vi "Add Signals.vi"(0 "reference in":refnum<class "SigMath.lvclass">, 5 "error in (no error)":errorcluster, 7 "Select Signals":i32[](listbox)) -> (14 "reference out":refnum<class "SigMath.lvclass">, 19 "error out":errorcluster)   [LabVIEW 2020, in "SigMath.lvclass"]
uses:
  SigMath.lvclass
  API/GSwFormDSP_class/functions/Attribute List.ctl
  API/GSwFormDSP_class/functions/Attribute Options.ctl
  API/GSwFormDSP_class/GSwFormDSP.lvclass
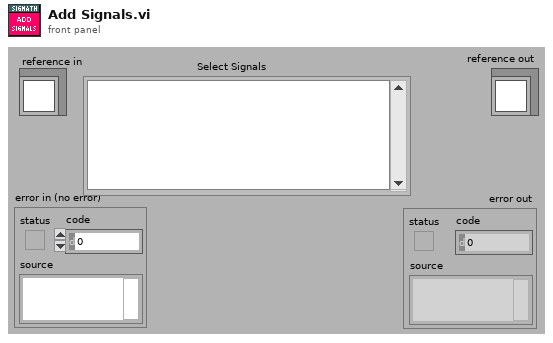
[diagram p1: front panel]
types:
  T1 = typedef "GSwFormDSP.lvclass/Attribute Options.ctl" = enum16{"Append to Attribute using \"( )\"", "Replace Attribute Value"}
  T2 = typedef "GSwFormDSP.lvclass/Attribute List.ctl" = string
  T3 = typedef "SigMath.lvclass/ObjectAttributes.ctl" = cluster{"SigMath Data":T4, "User CTRL Refs":T5}
  T4 = typedef "SigMath.lvclass/SigMath Data.ctl" = cluster{"New Time Data Obj?":bool, "GSwFormDSP":refnum<class "GSwFormDSP.lvclass">}
  T5 = typedef "SigMath.lvclass/SigMath User CTRL Refs.ctl" = cluster{"wForms":refnum<vi>, "Results wForms":refnum<vi>}
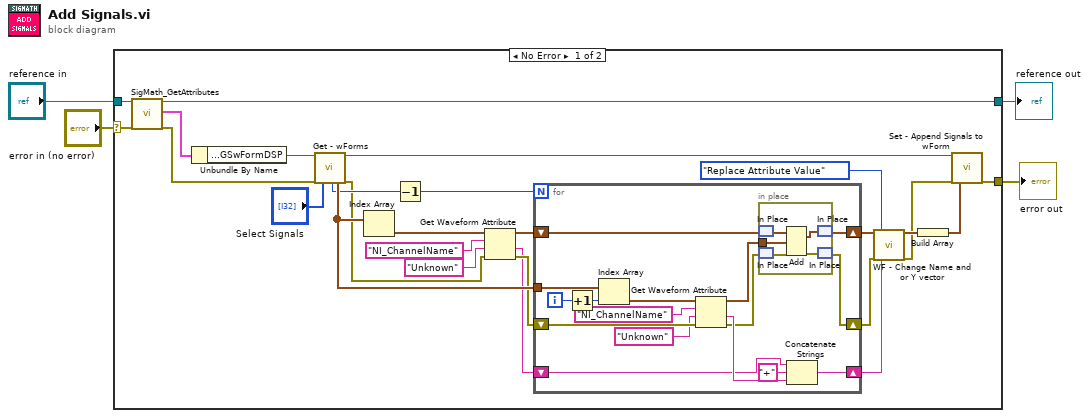
[diagram p0: block diagram]
diagram:
  n1 = case shown="No Error" "error in (no error)" {
    selector: "error in (no error)" -> [w30 w53]
    tunnel: [w20 w53] -> w3
    tunnel: [w29 w52] -> w1
    tunnel: "reference in" -> [w28 w52]
    frame No Error {
      n2 = call "SigMath_GetAttributes.vi"("reference in"=w28, "error in (no error)"=w30) -> ("reference out"=w29:refnum<class "SigMath.lvclass">, "attributes"=w27:T3, "error out"=w22:errorcluster)  [unwired: 14 in, 1 out]
      n3 = Unbundle By Name(w27) -> ("SigMath Data.GSwFormDSP"=w21:refnum<class "GSwFormDSP.lvclass">)
      n4 = call-dynamic "Get - wForms.vi"("reference in"=w21, "error in (no error)"=w22, "Indexes (Empty = ALL)"="Select Signals") -> ("Nb Signals"=w24:i32, "wForms"=w26:waveform(dbl)[], "reference out"=w19:refnum<class "GSwFormDSP.lvclass">, "error out"=w13:errorcluster)  [unwired: 13 in]
      n5 = Index Array(array=w26) -> (element=w16:waveform(dbl))  [unwired: 1 in]
      n6 = Decrement(x=w24) -> (x-1=w25:i32)
      n7 = Get Waveform Attribute(4:w13, 5:"Unknown", 6:T2 "NI_ChannelName" ("Attribute List"), 7:w16) -> (0:w12:errorcluster, 1:w11:string, 3:w15:waveform(dbl))  [unwired: 1 out]
      n8 = for {
        N: w25 -> [_]
        shift-right: [w34] -> w10
        shift-left: w15 -> [w35]
        tunnel: w26 -> [w45]
        shift-right: [w31] -> w7
        shift-left: w12 -> [w42]
        shift-right: [w36] -> w6
        shift-left: w11 -> [w37]
        i -> [w46]
        n9 = Increment(x=w46) -> (x+1=w44:i32)
        n10 = Index Array(array=w45, index=w44) -> (element=w43:waveform(dbl))
        n11 = Get Waveform Attribute(4:w42, 5:"Unknown", 6:T2 "NI_ChannelName" ("Attribute List"), 7:w43) -> (0:w32:errorcluster, 1:w38:string, 3:w33:waveform(dbl))  [unwired: 1 out]
        n12 = in-place {
          in-place-border: w33 -> [w50]
          n13 = in-place-match #1(w35) -> (w51:waveform(dbl))
          n14 = in-place-match #2(w32) -> (w49:errorcluster)
          n15 = Add(1:w50, 2:w51, 4:w49) -> (0:w48:waveform(dbl), 3:w47:errorcluster)
          n16 = in-place-match #1(w48) -> (w34:waveform(dbl))
          n17 = in-place-match #2(w47) -> (w31:errorcluster)
        }
        n18 = Concatenate Strings(w37, "+" ("string"), w38) -> (w36:string)
      }
      n19 = call "WF - Change Name and or Y vector.vi"("wForm IN"=w10, "error in (no error)"=w7, "Attribute Option"=Attribute_Options."Replace Attribute Value", "SigName Update"=w6) -> ("wForm OUT"=w9:waveform(dbl), "error out"=w5:errorcluster)  [unwired: 14 in]
      n20 = Build Array(w9) -> (w18:waveform(dbl)[])
      n21 = call "Set - Append Signals to wForm.vi"("reference in"=w19, "error in (no error)"=w5, "New Signals"=w18) -> ("error out"=w20:errorcluster)  [unwired: 15 in, 1 out]
    }
    frame Error {
    }
  }
  "error out" <- w3
  "reference out" <- w1
